vi "Reshape ICCD Parameters Table Row.vi"(8 "error in (no error)":errorcluster, 10 "Header":string[](array[string]), 11 "Array in":string[](array[string])) -> (0 "error out":errorcluster, 2 "Header out":string[](array[string]), 3 "Array out":string[][](array[string]))   [LabVIEW 2021, in "AlliGator Camera Noise Influence on Lifetime.lvlib"]
uses:
  AlliGator Camera Noise Influence on Lifetime.lvlib
  Strings/Strings.lvlib
panel:
  out "exponent":i32[](array[numeric])
  out "prefactor":i32[](array[numeric])
  out "MCP":i32[](array[numeric])
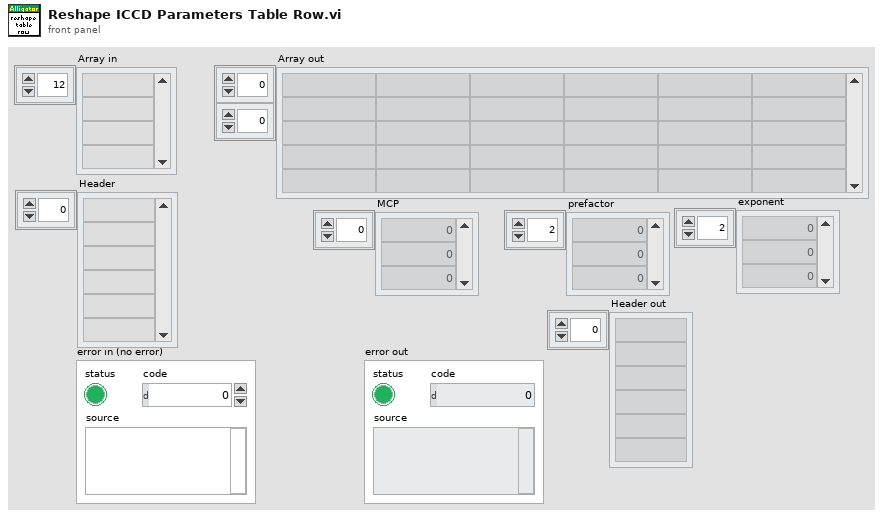
[diagram p1: front panel]
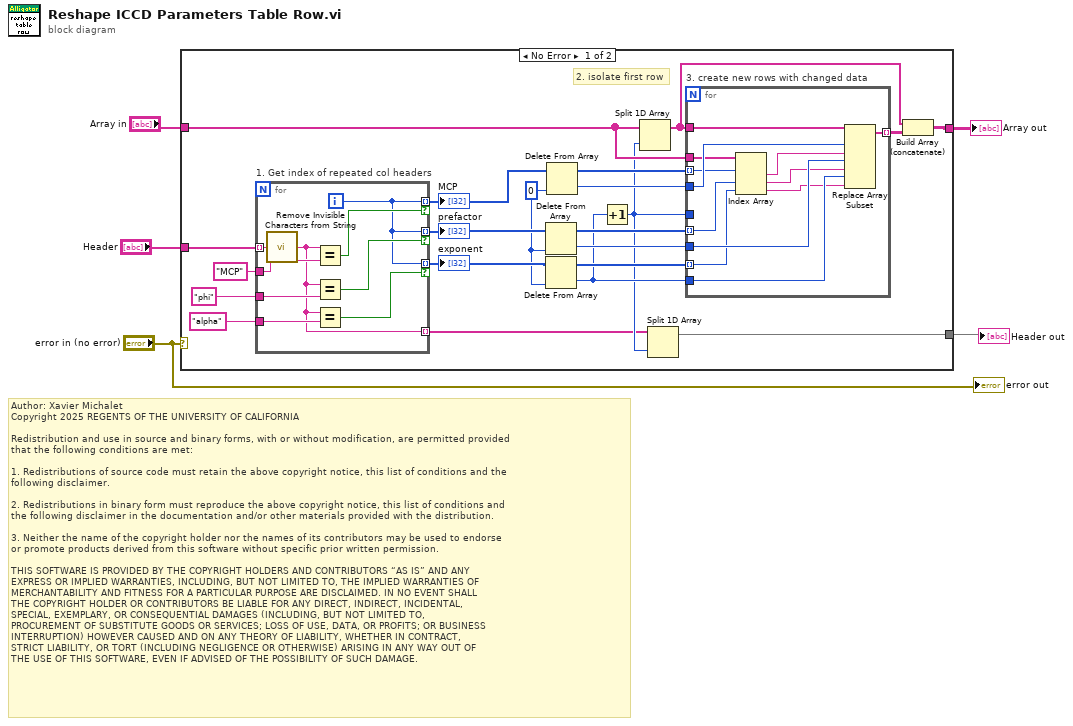
[diagram p0: block diagram]
diagram:
  # "Author: Xavier Michalet\nCopyright 2025 REGENTS OF THE UNIVERSITY OF CALIFORNIA\n\nRedistribution and use in source and binary forms, with or without modification, are permitted provided\nthat the following conditions are met:\n\n1. Redistributions of source code must retain the above copyright notice, this list of conditions and the\nfollowing disclaimer.\n\n2. Redistributions in binary form must reproduce the above copyright notice, this list of conditions and\nthe following disclaimer in the documentation and/or other materials provided with the distribution.\n\n3. Neither the name of the copyright holder nor the names of its contributors may be used to endorse \nor promote products derived from this software without specific prior written permission.\n\nTHIS SOFTWARE IS PROVIDED BY THE COPYRIGHT HOLDERS AND CONTRIBUTORS “AS IS” AND ANY \nEXPRESS OR IMPLIED WARRANTIES, INCLUDING, BUT NOT LIMITED TO, THE IMPLIED WARRANTIES OF\nMERCHANTABILITY AND FITNESS FOR A PARTICULAR PURPOSE ARE DISCLAIMED. IN NO EVENT SHALL\nTHE COPYRIGHT HOLDER OR CONTRIBUTORS BE LIABLE FOR ANY DIRECT, INDIRECT, INCIDENTAL, \nSPECIAL, EXEMPLARY, OR CONSEQUENTIAL DAMAGES (INCLUDING, BUT NOT LIMITED TO, \nPROCUREMENT OF SUBSTITUTE GOODS OR SERVICES; LOSS OF USE, DATA, OR PROFITS; OR BUSINESS\nINTERRUPTION) HOWEVER CAUSED AND ON ANY THEORY OF LIABILITY, WHETHER IN CONTRACT, \nSTRICT LIABILITY, OR TORT (INCLUDING NEGLIGENCE OR OTHERWISE) ARISING IN ANY WAY OUT OF\nTHE USE OF THIS SOFTWARE, EVEN IF ADVISED OF THE POSSIBILITY OF SUCH DAMAGE."
  n1 = case shown="No Error" "error in (no error)" {
    tunnel: "Header" -> [w8 w48]
    tunnel: "Array in" -> [w13 _]
    tunnel: [w10 _] -> w3
    tunnel: [w7 w48] -> w1
    frame No Error {
      w20 = 0 ("index")
      # "2. isolate first row"
      n2 = for "1. Get index of repeated col headers" {
        tunnel: w8 -> [w42] mode=indexing
        tunnel: "MCP" ("header") -> [w47]
        tunnel: [w41] -> w23 mode=indexing if=w46
        tunnel: "phi" ("header") -> [w45]
        tunnel: [w41] -> w22 mode=indexing if=w44
        tunnel: "alpha" ("header") -> [w43]
        tunnel: [w41] -> w21 mode=indexing if=w40
        tunnel: [w39] -> w6 mode=indexing
        i -> [w41]
        n3 = call "Remove Invisible Characters from String.vi"("String"=w42) -> ("result string"=w39:string)  [unwired: 3 in]
        n4 = Equal?(x=w39, y=w47) -> (x = y?=w46:bool)
        n5 = Equal?(x=w39, y=w45) -> (x = y?=w44:bool)
        n6 = Equal?(x=w39, y=w43) -> (x = y?=w40:bool)
      }
      "MCP" <- w23
      "prefactor" <- w22
      "exponent" <- w21
      n7 = Delete From Array(array=w22, index=w20) -> (deleted portion=w15:i32, array with subset deleted=w18:i32[])  [unwired: 1 in]
      n8 = Delete From Array(array=w21, index=w20) -> (deleted portion=w14:i32, array with subset deleted=w17:i32[])  [unwired: 1 in]
      n9 = Delete From Array(array=w23, index=w20) -> (deleted portion=w16:i32, array with subset deleted=w19:i32[])  [unwired: 1 in]
      n10 = Increment(x=w14) -> (x+1=w9:i32)
      n11 = Split 1D Array(array=w13, index=w9) -> (first subarray=w11:string[])  [unwired: 1 out]
      n12 = Split 1D Array(array=w6, index=w9) -> (first subarray=w7:string[])  [unwired: 1 out]
      n13 = for "3. create new rows with changed data" {
        tunnel: w11 -> [w38]
        tunnel: w19 -> [w33] mode=indexing
        tunnel: w18 -> [w32] mode=indexing
        tunnel: w17 -> [w31] mode=indexing
        tunnel: w16 -> [w37]
        tunnel: w15 -> [w36]
        tunnel: w14 -> [w35]
        tunnel: w13 -> [w34]
        tunnel: [w27] -> w12 mode=indexing
        tunnel: w9 -> [_]
        n14 = Index Array(array=w34, index #1=w33, index #2=w32, index #3=w31) -> (element #1=w30:string, element #2=w29:string, element #3=w28:string)
        n15 = Replace Array Subset(array=w38, new element #1=w30, index #1=w37, new element #2=w29, index #2=w36, new element #3=w28, index #3=w35) -> (w27:string[])
      }
      n16 = Build Array (concatenate)(w11, w12) -> (w10:string[][])
    }
    frame Error {
    }
  }
  "Array out" <- w3
  "Header out" <- w1
  "error out" <- "error in (no error)"
